vi "Reset Waveforms.vi"(8 "error in (no error)":errorcluster, 11 "Model in":refnum<class "Model.lvclass">) -> (0 "error out":errorcluster, 3 "Model out":refnum<class "Model.lvclass">)   [LabVIEW 2015, in "Model.lvclass"]
uses:
  Model.lvclass
  Model.lvclass/Model.ctl
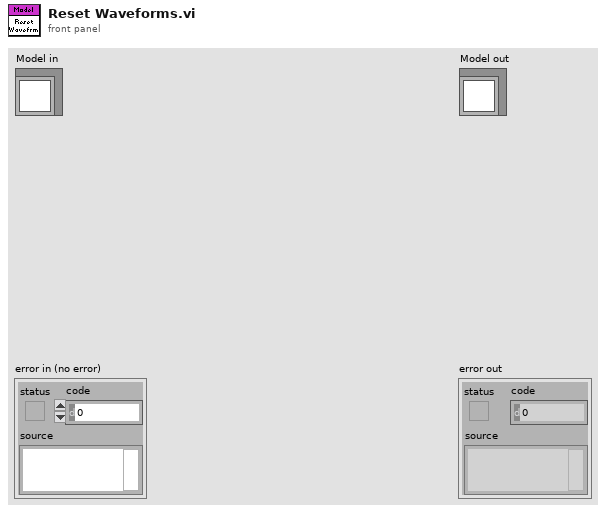
[diagram p1: front panel]
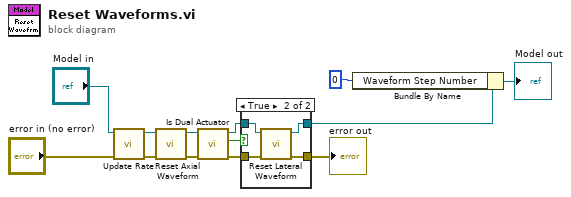
[diagram p0: block diagram]
diagram:
  n1 = call "Update Rate.vi"("error in (no error)"="error in (no error)", "Model in"="Model in") -> ("error out"=w8:errorcluster, "Model out"=w7:refnum<class "Model.lvclass">)  [unwired: 8 in]
  n2 = call "Reset Axial Waveform.vi"("error in (no error)"=w8, "Model in"=w7) -> ("error out"=w1:errorcluster, "Model out"=w5:refnum<class "Model.lvclass">)  [unwired: 8 in]
  n3 = call "Is Dual Actuator.vi"("error in (no error)"=w1, "Model in"=w5) -> ("error out"=w2:errorcluster, "Is Dual Actuator"=w3:bool, "Model out"=w4:refnum<class "Model.lvclass">)  [unwired: 7 in]
  n4 = case shown="True" w3 {
    tunnel: w4 -> [w15 w19]
    tunnel: [w15 w18] -> w11
    tunnel: w2 -> [w14 w17]
    tunnel: [w14 w16] -> w10
    frame False {
    }
    frame True {
      n5 = call "Reset Lateral Waveform.vi"("error in (no error)"=w17, "Model in"=w19) -> ("error out"=w16:errorcluster, "Model out"=w18:refnum<class "Model.lvclass">)  [unwired: 8 in]
    }
  }
  "error out" <- w10
  n6 = Bundle By Name(cluster=w11, "Waveform Step Number"=u16 0) -> (→"Model out":refnum<class "Model.lvclass">)
